vi "Multi_09_65.vi"() -> ()   [LabVIEW 2015]
uses:
  x64/Debug/BERTTA.dll
panel:
  in  "Numeric 19":dbl
  in  "Numeric 9":dbl
  in  "DAQ 9217 (PT100) 2":errorcluster
  out "element":bool
  out "Started:":string
  in  "SHUTDOWN":bool
  in  "MASTER CONTROL":bool
  in  "Tab Control":T1(tab)
  in  "Read Seq":bool
  in  "Save Seq":bool
  in  "Configuration file":path=path "C:/Users/shresplab/Desktop/BerttaConfiguration.lvm" caption="Filename"
  in  "OK Button 2":bool
  out "Boolean":bool
  in  "User (initials)":string
  in  "Project name":string
  in  "Description":string
  out "Output file":string
  out "RPM":dbl
  out "Torque":dbl
  out "Tj out":dbl
  out "Tj in":dbl
  out "T set":dbl
  out "Current step":i32
  out "PUMP1":bool
  out "Target amount":dbl
  out "Scale weight":dbl
  out "Amount now":dbl
  out "Flow rate":dbl
  out "Time to target":dbl format="%<%H:%M:%S>t"
  out "Current step":dbl
  out "Target":dbl
  out "Amount now":dbl
  out "Amount now":dbl
  out "Target":dbl
  out "Current step":dbl
  out "Time to target":dbl format="%<%H:%M:%S>t"
  out "Flow rate":dbl
  out "Amount now":dbl
  out "Scale weight":dbl
  out "Target amount":dbl
  out "PUMP2":bool
  out "Sensor OK 6":bool
  out "Sensor OK 5":bool
  out "Sensor OK 4":bool
  out "Sensor OK 3":bool
  in  "OK Button":bool
  in  "Add comment":string
  out "Tr":dbl
  out "Tj in":dbl
  out "Tj out":dbl
  out "T set":dbl
  out "Current step":i32
  out "RPM":dbl
  out "Torque":dbl
  out "Waveform Chart 5":dynamicdata(graph)
  out "Waveform Chart 6":dynamicdata(graph)
  out "Waveform Chart 7":dynamicdata(graph)
  out "Sensor OK 7":bool
  out "Sensor OK 8":bool
  out "Sensor OK 9":bool
  out "Sensor OK 10":bool
  in  "Tab Control 2":T2(tab)
  out "Waveform Chart 3":dynamicdata(graph)
  out "Waveform Chart 8":dynamicdata(graph)
  out "Waveform Chart 11":dynamicdata(graph)
  out "Waveform Chart 9":dynamicdata(graph)
  out "Waveform Chart 16":dynamicdata(graph)
  out "Table":string[][](table)=[["14.8.2017 18.06.59", "0,000000", "417,670000", "-0,150000", "1,000000", "22,220000", "23,366837", "23,574959", "23,985852", "23,690000", "240,000000", "4,000000", "0,000000", "397,000000", "-397,000000", "1,000000"], ["14.8.2017 18.07.06", "0,000000", "417,640000", "-0,120000", "1,000000", "22,220000", "23,763115", "23,906257", "23,985694", "23,680000", "240,000000", "4,000000", "0,000000", "397,000000", "-397,000000", "1,000000"], ["14.8.2017 18.07.13", "0,000000", "417,640000", "-0,120000", "1,000000", "22,220000", "23,965922", "24,013440", "23,984906", "23,670000", "240,000000", "4,100000", "3,000000", "397,000000", "-397,000000", "1,000000"], ["14.8.2017 18.07.21", "0,000000", "417,640000", "-0,120000", "1,000000", "22,220000", "23,943860", "23,900110", "23,987113", "23,670000", "240,000000", "4,000000", "0,000000", "397,000000", "-397,000000", "1,000000"], ["14.8.2017 18.07.28", "0,000000", "417,640000", "-0,120000", "1,000000", "22,220000", "23,736328", "23,600018", "23,989004", "23,660000", "240,000000", "4,000000", "0,000000", "397,000000", "-397,000000", "1,000000"], ["14.8.2017 18.07.36", "0,000000", "417,640000", "-0,120000", "1,000000", "22,220000", "23,480910", "23,324538", "23,991053", "23,660000", "240,000000", "4,000000", "0,000000", "397,000000", "-397,000000", "1,000000"], ["14.8.2017 18.07.43", "0,000000", "417,640000", "-0,120000", "2,000000", "22,220000", "23,195579", "23,008270", "23,999093", "23,650000", "240,000000", "4,000000", "0,000000", "397,000000", "-397,000000", "1,000000"], ["14.8.2017 18.07.51", "0,000000", "417,650000", "-417,650000", "1,000000", "22,220000", "22,862541", "22,649021", "24,003979", "23,650000", "240,000000", "4,000000", "0,000000", "397,000000", "-397,000000", "2,000000"], ["14.8.2017 18.07.58", "0,000000", "417,640000", "0,010000", "1,000000", "22,220000", "22,541353", "22,354878", "24,005398", "23,650000", "240,000000", "4,000000", "0,000000", "397,000000", "-397,000000", "1,000000"], ["14.8.2017 18.08.06", "0,000000", "417,640000", "0,010000", "1,000000", "22,220000", "22,347931", "22,253738", "24,007605", "23,640000", "240,000000", "4,100000", "0,000000", "397,000000", "-397,000000", "1,000000"], ["14.8.2017 18.08.13", "0,000000", "417,640000", "0,010000", "1,000000", "22,220000", "22,329030", "22,302102", "24,006028", "23,640000", "240,000000", "4,000000", "0,000000", "395,820000", "-395,820000", "1,000000"], ["14.8.2017 18.08.20", "0,000000", "417,640000", "0,010000", "1,000000", "22,220000", "22,466849", "22,511320", "24,002403", "23,630000", "240,000000", "4,000000", "0,000000", "395,830000", "-0,010000", "1,000000"], ["14.8.2017 18.08.28", "0,000000", "417,640000", "0,010000", "1,000000", "22,220000", "22,707062", "22,835101", "24,000984", "23,620000", "240,000000", "4,000000", "0,000000", "395,830000", "-0,010000", "1,000000"], ["14.8.2017 18.08.35", "0,000000", "417,640000", "0,010000", "1,000000", "22,220000", "23,054104", "23,232979", "24,001299", "23,600000", "240,000000", "4,000000", "0,000000", "395,830000", "-0,010000", "1,000000"], ["14.8.2017 18.08.43", "0,000000", "417,640000", "0,010000", "1,000000", "22,220000", "23,412371", "23,522793", "24,002560", "23,590000", "240,000000", "4,000000", "0,000000", "395,820000", "0,000000", "1,000000"], ["14.8.2017 18.08.51", "0,000000", "417,640000", "0,010000", "1,000000", "22,220000", "23,596247", "23,656125", "24,003821", "23,580000", "240,000000", "4,000000", "0,000000", "395,820000", "0,000000", "1,000000"]]
  in  "Reset":bool
  in  "Numeric 4":dbl=20.0
  in  "Numeric 3":dbl=30.0
  in  "Numeric 2":dbl=40.0
  in  "Numeric 1":dbl=30.0
  in  "Numeric":dbl=20.0
  out "LED5":bool
  out "LED4":bool
  out "LED3":bool
  out "LED2":bool
  out "LED1":bool
  out "LED6":bool
  in  "Numeric 5":dbl=5.0
  in  "Numeric 6":dbl=5.0
  in  "Numeric 7":dbl=5.0
  in  "Numeric 8":dbl=5.0
  in  "T ext / T ext 2":enum32{"External 1", "External 2"}(radio)
  out "Sensor OK":bool
  in  "T fail":dbl=20.0
  in  "?":bool
  in  "T manual setpoint":dbl=20.0
  in  "Lauda port":dbl=1.0
  in  "Manual select":enum32{"Tr", "Tj"}(radio)
  in  "PAUSE":bool
  out "Waveform Chart":dynamicdata(graph)
  out "T external 2":dbl
  in  "Reset 2":bool
  in  "Numeric 18":dbl=20.0
  in  "Numeric 17":dbl=30.0
  in  "Numeric 16":dbl=40.0
  in  "Numeric 15":dbl=30.0
  in  "Numeric 14":dbl=20.0
  out "Boolean 13":bool
  out "Boolean 11":bool
  out "Boolean 10":bool
  out "Boolean 9":bool
  out "Boolean 8":bool
  out "Boolean 20":bool
  in  "Numeric 13":dbl=5.0
  in  "Numeric 12":dbl=5.0
  in  "Numeric 11":dbl=5.0
  in  "Numeric 10":dbl=5.0
  in  "T ext / T ext 3":enum32{"External 1", "External 2"}(radio)
  out "Sensor OK 2":bool
  in  "T fail":dbl=20.0
  in  "?":bool
  in  "T manual setpoint":dbl=20.0
  in  "Lauda port":dbl=2.0
  in  "Manual select 2":enum32{"Tr", "Tj"}(radio)
  in  "PAUSE 2":bool
  out "Waveform Chart 2":dynamicdata(graph)
  out "T external 2":dbl
  out "Led11 5":bool
  in  "Port":i32=7
  in  "Radio Buttons 4":enum32{"Reglo Digital", "Reglo Analog", "PAM"}(radio)
  out "Speed":dbl
  out "mA":dbl format="%#_2g"
  in  "Port":i32=6
  out "RPM":dbl format="%_4f"
  out "Led10 3":bool
  out "Led9 3":bool
  out "Led8 3":bool
  out "Led7 3":bool
  out "Led6 3":bool
  out "Led5 3":bool
  out "Led4 3":bool
  out "Led3 3":bool
  out "Led2 3":bool
  out "Led1 3":bool
  in  "PumpSeq 4":dbl[][](array[numeric])=[[1.0, 1.0, 7.0], [2.0, 1.0, 2.0], [3.0, 1.0, 100.0], [0.0, 0.0, 0.0], [0.0, 0.0, 0.0], [0.0, 0.0, 0.0], [0.0, 0.0, 0.0], [0.0, 0.0, 0.0], [0.0, 0.0, 0.0], [0.0, 0.0, 0.0], [0.0, 1.0, 0.0]]
  in  "?":bool
  out "Flow rate (g/min)":dbl
  out "Scale reading":dbl
  out "Step amount now":dbl
  in  "Grams / min":dbl
  out "Waveform Chart 14":dynamicdata(graph)
  in  "?":bool
  out "Total amount now":dbl
  out "Total time 4":dbl
  out "Total amount target 4":dbl
  out "Led11 4":bool
  in  "Reset 5":bool
  out "Elapsed / step":i32
  out "Time to target":dbl format="%<%H:%M:%S>t"
  out "Led11":bool
  in  "Port":i32=9
  in  "Radio Buttons 2":enum32{"Reglo Digital", "Reglo Analog", "PAM"}(radio)
  out "Speed":dbl
  out "mA":dbl format="%#_2g"
  in  "Port":i32=8
  out "RPM":dbl format="%_4f"
  out "Led10":bool
  out "Led9":bool
  out "Led8":bool
  out "Led7":bool
  out "Led6":bool
  out "Led5":bool
  out "Led4":bool
  out "Led3":bool
  out "Led2":bool
  out "Led1":bool
  in  "PumpSeq 2":dbl[][](array[numeric])=[[1.0, 1.0, 7.0], [2.0, 1.0, 2.0], [3.0, 1.0, 100.0], [0.0, 0.0, 0.0], [0.0, 0.0, 0.0], [0.0, 0.0, 0.0], [0.0, 0.0, 0.0], [0.0, 0.0, 0.0], [0.0, 0.0, 0.0], [0.0, 0.0, 0.0], [0.0, 1.0, 0.0]]
  in  "?":bool
  out "Flow rate (g/min)":dbl
  out "Scale reading":dbl
  out "Step amount now":dbl
  in  "Grams / min":dbl
  out "Waveform Chart 10":dynamicdata(graph)
  in  "?":bool
  out "Total amount now":dbl
  out "Total time 2":dbl
  out "Total amount target 2":dbl
  out "Led11":bool
  in  "Reset 3":bool
  out "Elapsed / step":i32
  out "Time to target":dbl format="%<%H:%M:%S>t"
  in  "OK Button 3":bool
  in  "Port":dbl=10.0
  out "RPM":dbl
  out "Torque":dbl
  in  "Set RPM":dbl
  out "Waveform Chart 4":dynamicdata(graph)
  in  "Set RPM":dbl
  in  "Port":dbl=20.0
  out "RPM":dbl
  out "Torque":dbl
  in  "OK Button 4":bool
  out "Waveform Chart 15":dynamicdata(graph)
  in  "Treshold (T/C) Lauda 2":dbl=0.5
  in  "Treshold (T/C) Lauda 1":dbl=0.5
  out "DAQ 9217 (PT100)":errorcluster
  # "PUMP & SCALE 1"
  # "STEP"
  # "TOTAL"
  # "PUMP & SCALE 2"
  # "STEP"
  # "TOTAL"
  # "Manual control"
  # "Secondary temperature sensor"
  # "Device communication"
  # "Temp"
  # "Time"
  # "Manual control"
  # "Secondary temperature sensor"
  # "Device communication"
  # "Temp"
  # "Time"
  # "Grams    /   min"
  # "End of sequence"
  # "Manual control"
  # "Device communication"
  # "Pump configuration"
  # "Scale configuration"
  # "SCALE 1"
  # "Grams    /   min"
  # "End of sequence"
  # "Manual control"
  # "Device communication"
  # "Pump configuration"
  # "Scale configuration"
  # "SCALE 2"
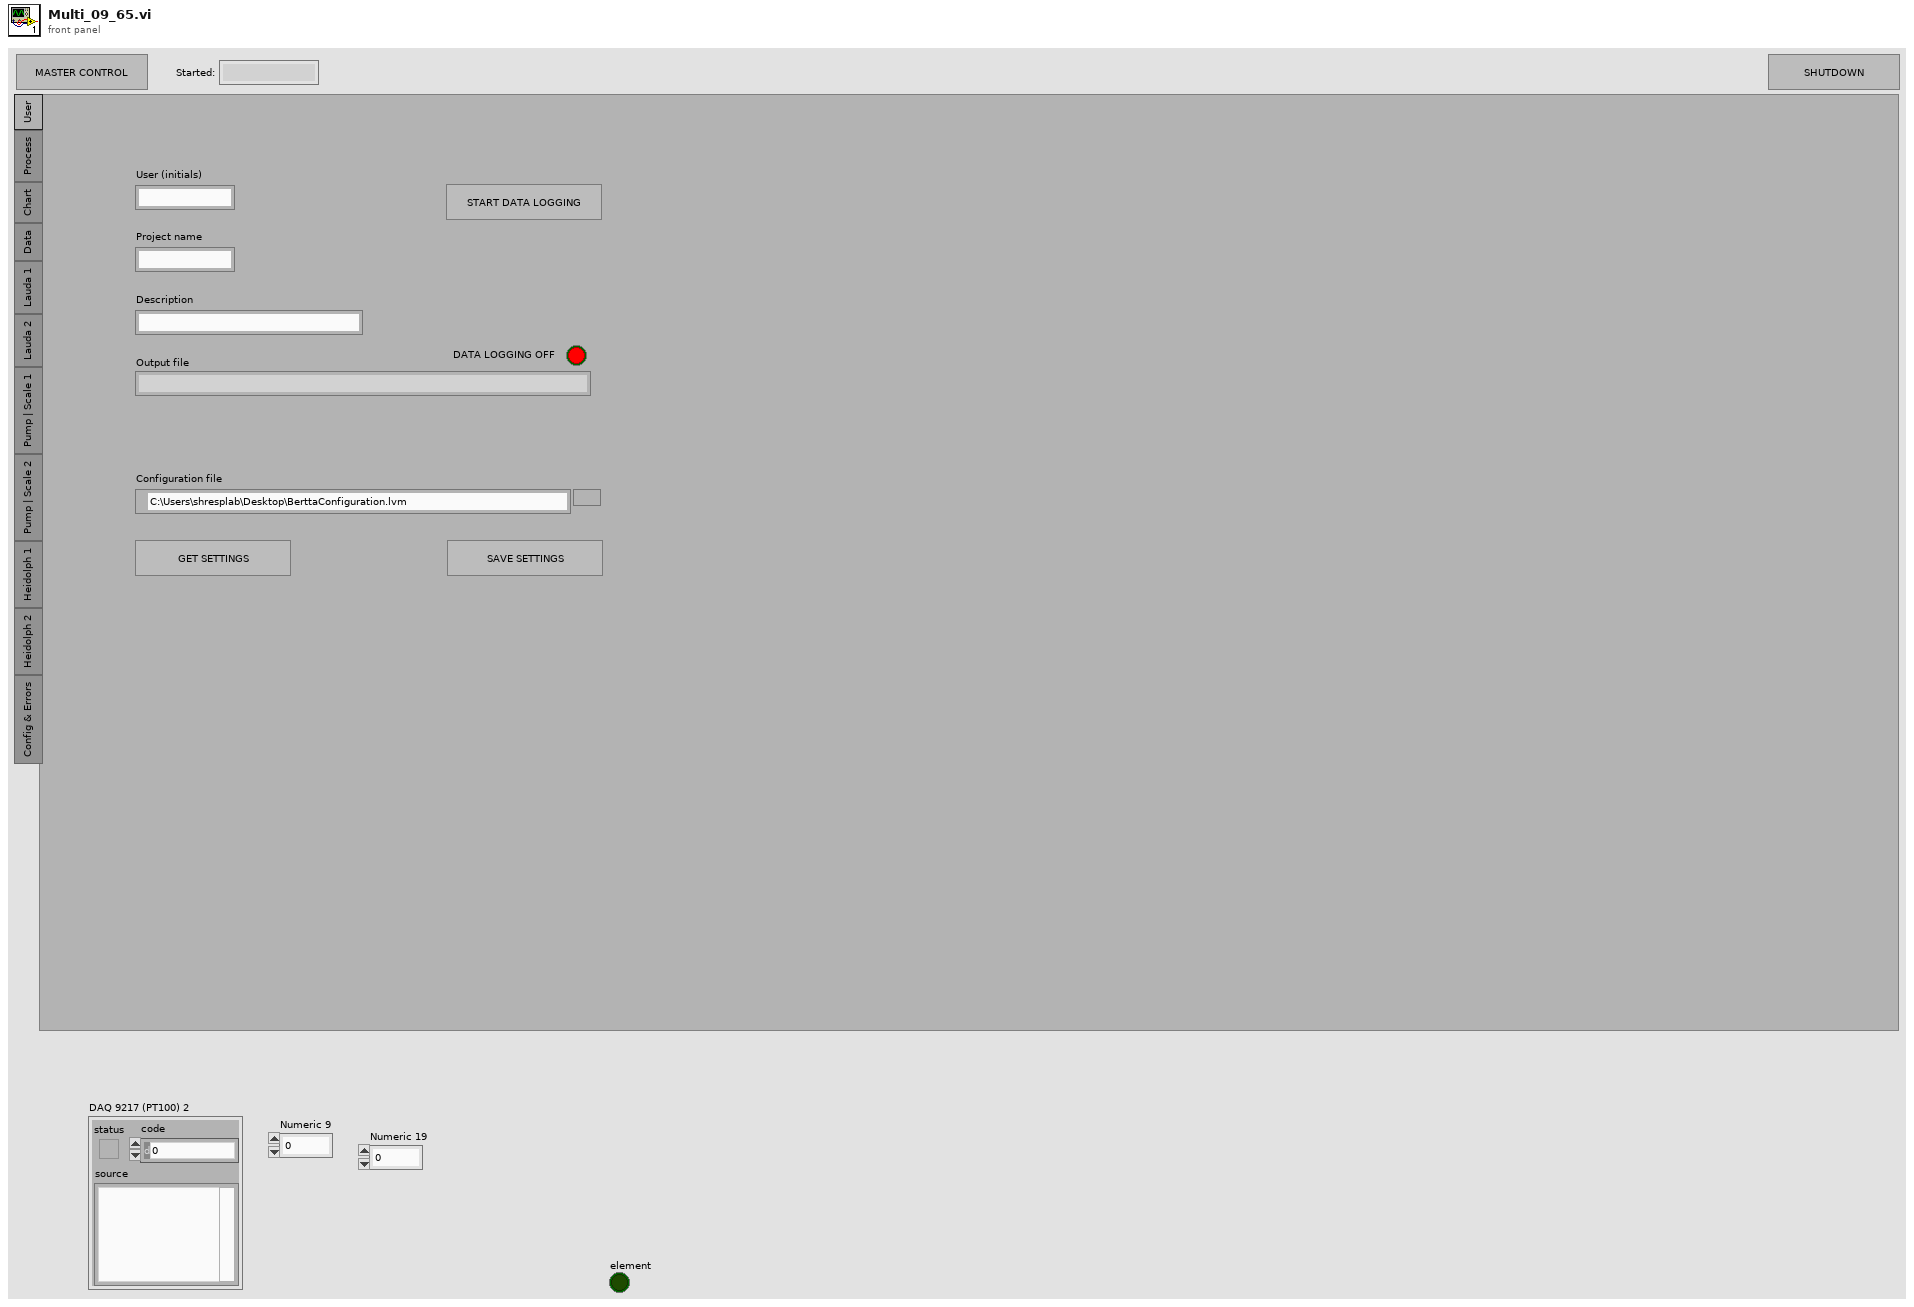
[diagram p1: front panel]
types:
  T1 = enum32{"User", "Process", "Chart", "Data", "Lauda 1", "Lauda 2", "Pump | Scale 1", "Pump | Scale 2", "Heidolph 1", "Heidolph 2", "Config & Errors"}
  T2 = enum32{"Temperatures", "Scale / Pump 1", "Scale / Pump 2", "RPM / Torque 1", "RPM / Torque 2"}
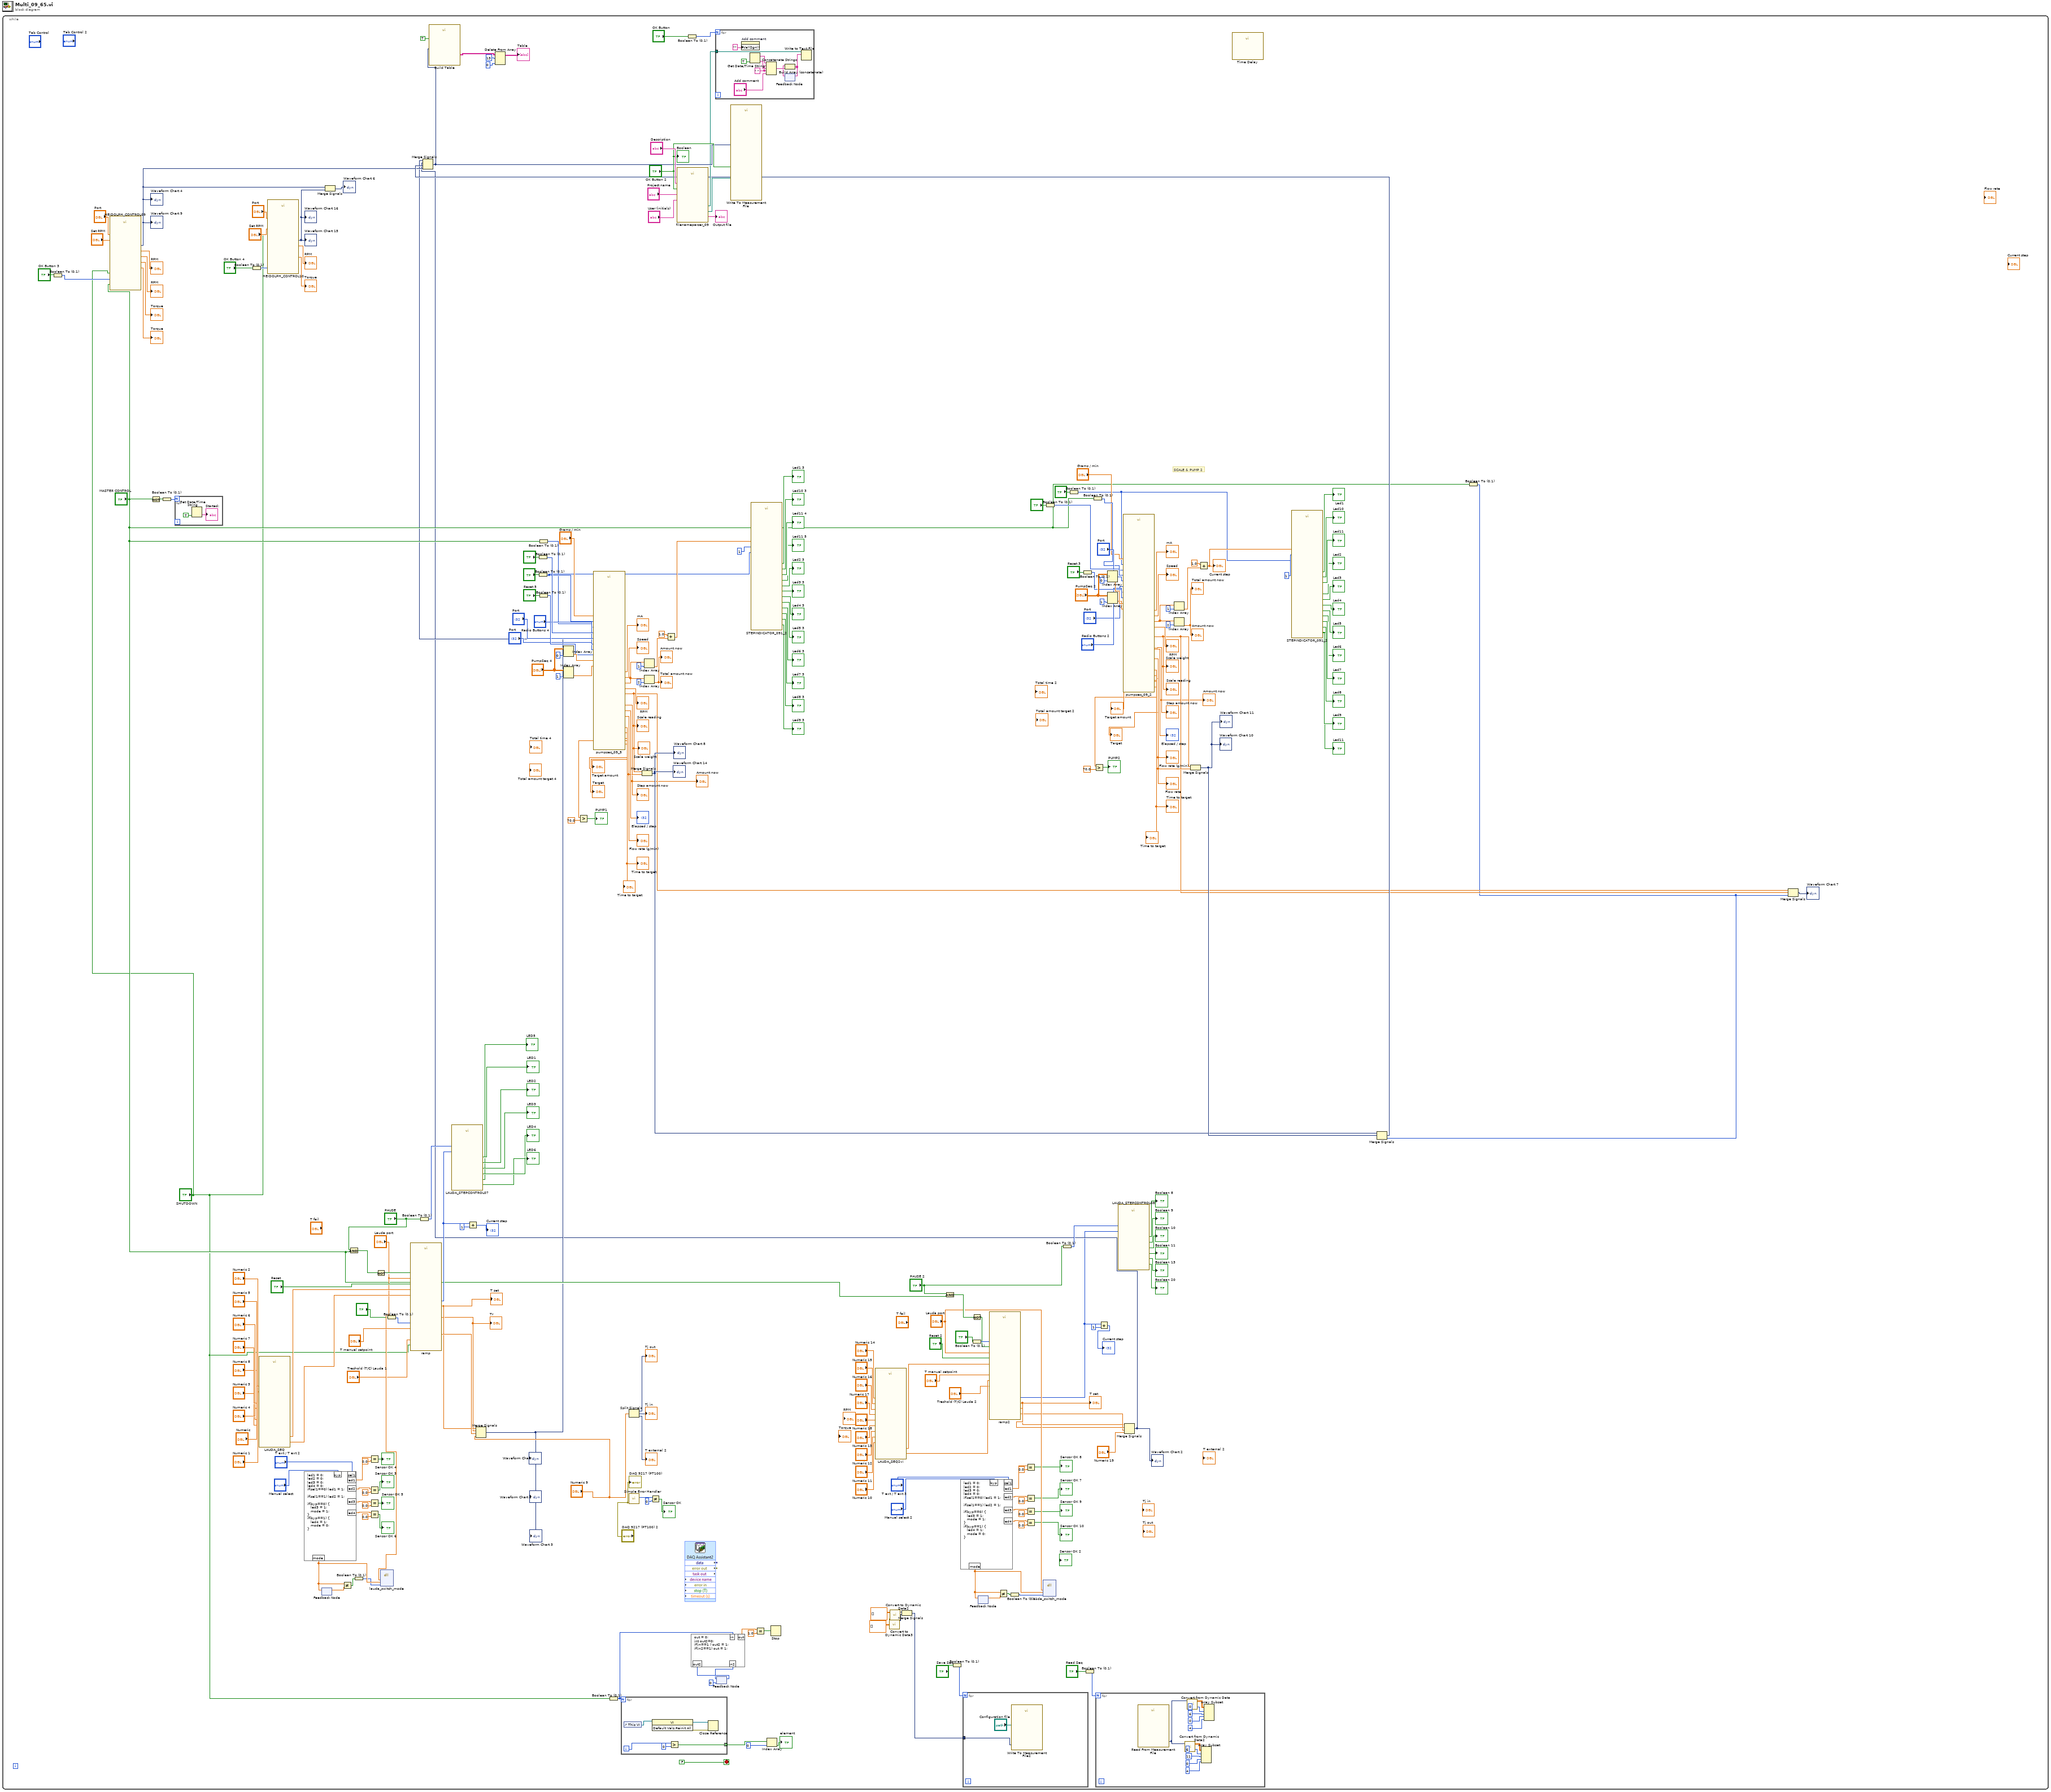
[diagram p0: block diagram]
diagram:
  n1 = while {
    stop <- FALSE stop-if-true
    # "SCALE & PUMP 2"
    n2 = Boolean To (0,1)(Boolean="OK Button 3") -> (0, 1=w5:i16)
    n3 = call "HEIDOLPH_CONTROL09.vi"("master"="MASTER CONTROL", "shutdown"="SHUTDOWN", "mode"=w5, "Set RPM"="Set RPM", "Device port"="Port") -> ("Dynamic Data"=w96:dynamicdata, "RPM"=→"RPM":dbl, "RPM 2"=→"RPM":dbl, "Torque"=→"Torque":dbl, "Torque 2"=→"Torque":dbl)  [unwired: 2 in]
    "Waveform Chart 4" <- w96
    "Waveform Chart 9" <- w96
    n4 = Not(x="MASTER CONTROL") -> (.not. x?=w253:bool)
    n5 = Boolean To (0,1)(Boolean=w253) -> (0, 1=w254:i16)
    n6 = for {
      N: w254 -> [_]
      n7 = Get Date/Time String(want seconds? (F)=TRUE) -> (time string=→"Started:":string)  [unwired: 2 in, 1 out]
    }
    n8 = Boolean To (0,1)(Boolean="OK Button 4") -> (0, 1=w3:i16)
    n9 = call "LAUDA_SEQ.vi"("Numeric 2"="Numeric 2", "Numeric 1"="Numeric 1", "Numeric"="Numeric", "Numeric 5"="Numeric 5", "Numeric 6"="Numeric 6", "Numeric 7"="Numeric 7", "Numeric 8"="Numeric 8", "Numeric 3"="Numeric 3", "Numeric 4"="Numeric 4") -> ("output array"=w155:dbl[], "output array 2"=w154:dbl[])  [unwired: 5 in]
    n10 = call "HEIDOLPH_CONTROL10.vi"("shutdown"="SHUTDOWN", "mode"=w3, "Set RPM"="Set RPM", "Device port"="Port") -> ("Dynamic Data"=w63:dynamicdata, "RPM"=→"RPM":dbl, "Torque"=→"Torque":dbl)  [unwired: 3 in, 2 out]
    "Waveform Chart 15" <- w63
    "Waveform Chart 16" <- w63
    n11 = formula code="led1 = 0;\nled2 = 0;\nled3 = 0;\nled4 = 0;\nif(sel1==0) led1 = 1;\n\nif(sel1==1) led2 = 1;\n\nif(byp==0) {\n   led3 = 1;\n   mode = 1;\n}\nif(byp==1) {\n   led4 = 1;\n   mode = 0;\n}"("sel1"="T ext / T ext 2", "byp"="Manual select") -> ("led1"=w224:dbl, "led2"=w222:dbl, "led3"=w217:dbl, "led4"=w216:dbl, "mode"=w149:dbl)
    n12 = feedback-in #1(w149) -> ()
    n13 = feedback #1() -> (w148:dbl)  [unwired: 1 in]
    n14 = Merge Signals(w96, w63) -> (→"Waveform Chart 6":dynamicdata)
    n15 = Not Equal?(x=w149, y=w148) -> (x != y?=w146:bool)
    n16 = And(x="PAUSE", y="MASTER CONTROL") -> (x .and. y?=w167:bool)
    n17 = Boolean To (0,1)(Boolean=w146) -> (0, 1=w147:i16)
    n18 = Equal?(x=w224, y=0.0) -> (x = y?=→"Sensor OK 4":bool)
    n19 = Equal?(x=w222, y=0.0) -> (x = y?=→"Sensor OK 3":bool)
    n20 = Equal?(x=w217, y=0.0) -> (x = y?=→"Sensor OK 5":bool)
    n21 = Equal?(x=w216, y=0.0) -> (x = y?=→"Sensor OK 6":bool)
    n22 = Not(x=w167) -> (.not. x?=w166:bool)
    n23 = dll-call lib="C:/Users/shresplab/OneDrive - Kemira Oyj/Documents/Visual Studio 2017/Projects/Bertta/BERTTA/x64/Debug/BERTTA.dll" fn="lauda_switch_mode"("port"="Lauda port", "mode"=w149, "enable"=w147) -> ()  [unwired: 7 in, 2 out]
    n24 = Boolean To (0,1)(Boolean="?") -> (0, 1=w152:i16)
    n25 = call "ramp.vi"("pause"=w166, "manual"=w152, "T_man"="T manual setpoint", "Seq"=w155, "reset"="Reset", "TimeParams"=w154, "shutdown"="SHUTDOWN", "port"="Lauda port", "treshold"="Treshold (T/C) Lauda 1") -> ("T in"=w95:dbl, "STEP"=w71:i32, "T ext"=w84:dbl, "T control"=w85:dbl)  [unwired: 2 in, 1 out]
    "Tr" <- w84
    "T set" <- w85
    n26 = Boolean To (0,1)(Boolean="PAUSE") -> (0, 1=w211:i16)
    n27 = call "LAUDA_STEPCONTROL07.vi"("step"=w71, "pause"=w211) -> ("LED6"=→"LED6":bool, "LED3"=→"LED3":bool, "LED2"=→"LED2":bool, "LED1"=→"LED1":bool, "LED4"=→"LED4":bool, "LED5"=→"LED5":bool)  [unwired: 4 in]
    n28 = Add(x=w71, y=1) -> (x+y=→"Current step":i32)
    n29 = Merge Signals(w85, w84, w95, "Numeric 9") -> (w13:dynamicdata)
    "Waveform Chart 3" <- w13
    "Waveform Chart" <- w13
    "Waveform Chart 5" <- w13
    n30 = Boolean To (0,1)(Boolean="?") -> (0, 1=w102:i16)
    n31 = Boolean To (0,1)(Boolean="?") -> (0, 1=w112:i16)
    n32 = Boolean To (0,1)(Boolean="MASTER CONTROL") -> (0, 1=w99:i16)
    n33 = Boolean To (0,1)(Boolean="Reset 5") -> (0, 1=w111:i16)
    n34 = Index Array(array="PumpSeq 4", index (col)=0) -> (element=w117:dbl[])  [unwired: 1 in]
    n35 = Index Array(array="PumpSeq 4", index (col)=1) -> (element=w139:dbl[])  [unwired: 1 in]
    n36 = call "pumpsec_09_5.vi"("reset"=w111, "master"=w99, "manual"=w102, "pause"=w112, "Port"="Port", "pump_type"="Radio Buttons 4", "port, Reglo D"="Port", "Target"=w117, "fr_manual"="Grams / min", "Time"=w139) -> ("pumpCtrl"=w80:dbl, "totaltarget"=→"Target":dbl, "target_step"=→"Target amount":dbl, "time_to_target"=→"Time to target" →"Time to target":dbl, "step_fr"=w94:dbl, "amount_step"=→"Amount now" →"Step amount now":dbl, "Reglo D"=→"RPM":dbl, "Scale"=w91:dbl, "mA"=→"mA":dbl, "elapsed_step"=→"Elapsed / step":dbl, "params"=w136:dbl[], "PAM"=→"Speed":dbl)  [unwired: 4 in, 2 out]
    "Scale weight" <- w91
    "Scale reading" <- w91
    "Flow rate (g/min)" <- w94
    n37 = Greater?(x=w80, y=70.0) -> (0:→"PUMP1":bool)
    n38 = Boolean To (0,1)(Boolean="SHUTDOWN") -> (0, 1=w229:i16)
    n39 = for {
      N: w229 -> [_]
      tunnel: [w296] -> w252 mode=indexing
      i -> [w298]
      n40 = control-ref of="This VI"() -> (w301:refnum<vi>)
      n41 = invoke class="VI" method="Default Vals.Reinit All"(reference=w301) -> (reference out=w299:refnum<vi>, error out=w300:errorcluster)  [unwired: 2 in, 1 out]
      n42 = Greater?(x=w298, y=0) -> (0:w296:bool)
      n43 = Close Reference(reference=w299, error in (no error)=w300) -> ()  [unwired: 1 out]
    }
    n44 = Split Signals("Numeric 9") -> (→"Tj out":dynamicdata, →"Tj in":dynamicdata, →"T external 2":dynamicdata)  [unwired: 3 in]
    n45 = call <vilib>:"Simple Error Handler.vi"("error in (no error)"="DAQ 9217 (PT100) 2") -> ("code out"=w262:i32)  [unwired: 4 in, 4 out]
    n46 = Merge Signals(w91, w94) -> (w98:dynamicdata)
    "Waveform Chart 8" <- w98
    "Waveform Chart 14" <- w98
    n47 = Index Array(array=w136, index=1) -> (element=w133:dbl)
    n48 = Index Array(array=w136, index=2) -> (element=→"Amount now" →"Total amount now":dbl)
    n49 = Not Equal?(x=w262, y=0) -> (x != y?=→"Sensor OK":bool)
    n50 = Add(x=1.0, y=w133) -> (x+y=w132:dbl)
    n51 = call "filenameparser_09.vi"("Description"="Description", "Project name"="Project name", "User (initials)"="User (initials)", "OK Button in"="OK Button 2") -> ("Output file"=→"Output file":string, "appended path 2"=w236:path, "appended path"=w235:path)  [unwired: 5 in]
    n52 = Boolean To (0,1)(Boolean="OK Button") -> (0, 1=w234:i16)
    n53 = for {
      N: w234 -> [_]
      tunnel: w235 -> [w275]
      w279 = " " ("string")
      n54 = property on="Add comment" class="Str"("Val(Sgnl)"="" ("Value (Signaling)")) -> ()  [unwired: 2 in, 2 out]
      n55 = Get Date/Time String(want seconds? (F)=TRUE) -> (date string=w282:string, time string=w280:string)  [unwired: 2 in]
      n56 = Concatenate Strings(w282, w279, w280, w279, "Add comment") -> (w278:string)
      n57 = feedback #2() -> (w277:string[])  [unwired: 1 in]
      n58 = Build Array (concatenate)(w277, w278) -> (w276:string[])
      n59 = feedback-in #2(w276) -> ()
      n60 = Write to Text File(file (use dialog)=w275, text=w276) -> ()  [unwired: 2 in, 3 out]
    }
    n61 = feedback #3(0) -> (w227:i32)
    n62 = formula code="out = 0;\nint out2=0;\nif(in==1 ) out2 = 1;\nif(in2==1) out = 1;"("in"=w229, "in2"=w227) -> ("out"=w231:dbl, "out2"=w228:i32)
    n63 = feedback-in #3(w228) -> ()
    n64 = call "STEPINDICATOR_091_2.vi"("current step"=w132, "enable"=i16 1, "manual"=w102) -> ("Led 8"=→"Led8 3":bool, "Led 10"=→"Led10 3":bool, "Led 11"=→"Led11 4":bool, "Led 7"=→"Led7 3":bool, "Led 1"=→"Led1 3":bool, "Led 6"=→"Led6 3":bool, "Led 2"=→"Led2 3":bool, "Led 12"=→"Led11 5":bool, "Led 5"=→"Led5 3":bool, "Led 4"=→"Led4 3":bool, "Led 3"=→"Led3 3":bool, "Led 9"=→"Led9 3":bool)  [unwired: 1 in]
    n65 = Equal?(x=w231, y=1.0) -> (x = y?=w230:bool)
    n66 = Index Array(array=w252, index=0) -> (element=→"element":bool)
    n67 = Stop(stop? (T)=w230) -> ()
    n68 = call "LAUDA_SEQ2vi.vi"("Numeric 2"="Numeric 16", "Numeric 1"="Numeric 15", "Numeric"="Numeric 14", "Numeric 5"="Numeric 13", "Numeric 6"="Numeric 12", "Numeric 7"="Numeric 11", "Numeric 8"="Numeric 10", "Numeric 3"="Numeric 17", "Numeric 4"="Numeric 18") -> ("output array"=w53:dbl[], "output array 2"=w52:dbl[])  [unwired: 5 in]
    n69 = call "Convert to Dynamic Data3"("2D Array"=dbl[][] []) -> ("Dynamic Data Type"=w213:dynamicdata)  [unwired: 3 in]
    n70 = call "Convert to Dynamic Data2"("2D Array"=dbl[][] []) -> ("Dynamic Data Type"=w250:dynamicdata)  [unwired: 3 in]
    n71 = Merge Signals(w250, w213) -> (w249:dynamicdata)
    n72 = And(x="PAUSE 2", y="MASTER CONTROL") -> (x .and. y?=w35:bool)
    n73 = Boolean To (0,1)(Boolean="Save Seq") -> (0, 1=w248:i16)
    n74 = formula code="led1 = 0;\nled2 = 0;\nled3 = 0;\nled4 = 0;\nif(sel1==0) led1 = 1;\n\nif(sel1==1) led2 = 1;\n\nif(byp==0) {\n   led3 = 1;\n   mode = 1;\n}\nif(byp==1) {\n   led4 = 1;\n   mode = 0;\n}"("sel1"="T ext / T ext 3", "byp"="Manual select 2") -> ("led1"=w40:dbl, "led2"=w49:dbl, "led3"=w46:dbl, "led4"=w45:dbl, "mode"=w22:dbl)
    n75 = for {
      N: w248 -> [_]
      tunnel: w249 -> [w295]
      n76 = call "Write To Measurement File2"("Signals"=w295, "Filename"="Configuration file") -> ()  [unwired: 15 in, 3 out]
    }
    n77 = Boolean To (0,1)(Boolean="?") -> (0, 1=w38:i16)
    n78 = Not(x=w35) -> (.not. x?=w34:bool)
    n79 = feedback #4() -> (w44:dbl)  [unwired: 1 in]
    n80 = feedback-in #4(w22) -> ()
    n81 = call "ramp2.vi"("pause"=w34, "manual"=w38, "T_man"="T manual setpoint", "Seq"=w53, "reset"="Reset 2", "TimeParams"=w52, "port"="Lauda port", "treshold"="Treshold (T/C) Lauda 2") -> ("T in"=w15:dbl, "STEP"=w9:i32, "T ext"=w16:dbl, "T control"=w11:dbl)  [unwired: 3 in, 1 out]
    "T set" <- w11
    n82 = Not Equal?(x=w22, y=w44) -> (x != y?=w43:bool)
    n83 = Boolean To (0,1)(Boolean=w43) -> (0, 1=w23:i16)
    n84 = Equal?(x=w40, y=0.0) -> (x = y?=→"Sensor OK 8":bool)
    n85 = Equal?(x=w49, y=0.0) -> (x = y?=→"Sensor OK 7":bool)
    n86 = Equal?(x=w46, y=0.0) -> (x = y?=→"Sensor OK 9":bool)
    n87 = Equal?(x=w45, y=0.0) -> (x = y?=→"Sensor OK 10":bool)
    n88 = dll-call lib="C:/Users/shresplab/OneDrive - Kemira Oyj/Documents/Visual Studio 2017/Projects/Bertta/BERTTA/x64/Debug/BERTTA.dll" fn="lauda_switch_mode"("port"="Lauda port", "mode"=w22, "enable"=w23) -> ()  [unwired: 7 in, 2 out]
    n89 = Boolean To (0,1)(Boolean="?") -> (0, 1=w200:i16)
    n90 = Boolean To (0,1)(Boolean="PAUSE 2") -> (0, 1=w31:i16)
    n91 = Boolean To (0,1)(Boolean="?") -> (0, 1=w141:i16)
    n92 = Boolean To (0,1)(Boolean="Reset 3") -> (0, 1=w197:i16)
    n93 = Boolean To (0,1)(Boolean="Read Seq") -> (0, 1=w245:i16)
    n94 = Boolean To (0,1)(Boolean="MASTER CONTROL") -> (0, 1=w191:i16)
    n95 = for {
      N: w245 -> [_]
      n96 = call "Read From Measurement File"() -> ("Signals"=w284:dynamicdata)  [unwired: 6 in, 5 out]
      n97 = call "Convert from Dynamic Data2"("Dynamic Data Type"=w284) -> ("Array"=w283:dbl[][])  [unwired: 3 in]
      n98 = call "Convert from Dynamic Data"("Dynamic Data Type"=w284) -> ("Array"=w291:dbl[][])  [unwired: 3 in]
      n99 = Array Subset(array=w283, index (row)=6 ("index"), length (row)=11 ("length"), index (col)=0 ("index"), length (col)=4 ("length")) -> ()  [unwired: 1 out]
      n100 = Array Subset(array=w291, index (row)=0 ("index"), length (row)=6 ("length"), index (col)=0 ("index"), length (col)=4 ("length")) -> ()  [unwired: 1 out]
    }
    n101 = Add(x=w9, y=1) -> (x+y=→"Current step":i32)
    n102 = Index Array(array="PumpSeq 2", index (col)=0 ("disabled index (col)")) -> (element=w203:dbl[])  [unwired: 1 in]
    n103 = Index Array(array="PumpSeq 2", index (col)=1 ("disabled index (col)")) -> (element=w202:dbl[])  [unwired: 1 in]
    n104 = call "LAUDA_STEPCONTROL08.vi"("step"=w9, "pause"=w31) -> ("LED6"=→"Boolean 20":bool, "LED3"=→"Boolean 10":bool, "LED2"=→"Boolean 9":bool, "LED1"=→"Boolean 8":bool, "LED4"=→"Boolean 11":bool, "LED5"=→"Boolean 13":bool)  [unwired: 4 in]
    n105 = call "pumpsec_09_2.vi"("reset"=w197, "master"=w191, "manual"=w141, "pause"=w200, "Port"="Port", "pump_type"="Radio Buttons 2", "port, Reglo D"="Port", "Target"=w203, "fr_manual"="Grams / min", "Time"=w202) -> ("pumpCtrl"=w76:dbl, "totaltarget"=→"Target":dbl, "target_step"=→"Target amount":dbl, "time_to_target"=→"Time to target" →"Time to target":dbl, "step_fr"=w93:dbl, "amount_step"=→"Amount now" →"Step amount now":dbl, "Reglo D"=→"RPM":dbl, "Scale"=w90:dbl, "mA"=→"mA":dbl, "elapsed_step"=→"Elapsed / step":dbl, "params"=w192:dbl[], "PAM"=→"Speed":dbl)  [unwired: 4 in, 2 out]
    "Scale weight" <- w90
    "Flow rate" <- w93
    "Scale reading" <- w90
    "Flow rate (g/min)" <- w93
    n106 = Greater?(x=w76, y=70.0) -> (0:→"PUMP2":bool)
    n107 = Merge Signals(w11, w16, w15, "Numeric 19") -> (w12:dynamicdata)
    "Waveform Chart 2" <- w12
    n108 = Index Array(array=w192, index=1) -> (element=w195:dbl)
    n109 = Index Array(array=w192, index=2) -> (element=→"Amount now" →"Total amount now":dbl)
    n110 = Merge Signals(w90, w93) -> (w100:dynamicdata)
    "Waveform Chart 11" <- w100
    "Waveform Chart 10" <- w100
    n111 = Add(x=1.0, y=w195) -> (x+y=w185:dbl)
    "Current step" <- w185
    n112 = call "Time Delay"() -> ()  [unwired: 11 in, 1 out]
    n113 = call "STEPINDICATOR_091_2.vi"("current step"=w185, "enable"=i16 1, "manual"=w141) -> ("Led 8"=→"Led8":bool, "Led 10"=→"Led10":bool, "Led 11"=→"Led11":bool, "Led 7"=→"Led7":bool, "Led 1"=→"Led1":bool, "Led 6"=→"Led6":bool, "Led 2"=→"Led2":bool, "Led 12"=→"Led11":bool, "Led 5"=→"Led5":bool, "Led 4"=→"Led4":bool, "Led 3"=→"Led3":bool, "Led 9"=→"Led9":bool)  [unwired: 1 in]
    n114 = Boolean To (0,1)(Boolean="MASTER CONTROL") -> (0, 1=w7:i16)
    n115 = Merge Signals(w98, w100, w7) -> (w97:dynamicdata)
    n116 = Merge Signals(w13, w12, w97, w96) -> (w241:dynamicdata)
    n117 = call "Build Table"("Include time data"=TRUE, "Signals"=w241) -> ("Table"=w240:string[][])  [unwired: 3 in, 6 out]
    n118 = Delete From Array(array=w240, length=13, index (col)=0 ("index (row)")) -> (array with subset deleted=→"Table":string[][])  [unwired: 1 in, 1 out]
    n119 = call "Write To Measurement File"("Signals"=w241, "Enable"="OK Button 2", "Filename"=w236) -> ()  [unwired: 14 in, 3 out]
    n120 = Merge Signals(w91, w90, w7) -> (→"Waveform Chart 7":dynamicdata)
    "DAQ 9217 (PT100)" <- "DAQ 9217 (PT100) 2"
    "Boolean" <- "OK Button 2"
  }
